vi "Check If Custom Device Enabled.vi"(8 "error in (no error)":errorcluster, 11 "Ballard ARINC 429 ref":T1 format="%.0x") -> (0 "error out":errorcluster, 2 "Is Custom Device Enabled?":bool, 3 "Ballard ARINC 429 ref":T1 format="%.0x")   [LabVIEW 2020, in "Ballard ARINC 429 Scripting.lvlib"]
doc: "Returns a boolean value that is <b>True</b> if the Ballard ARINC 429 custom device is <b>Enabled</b>, and <b>False</b> if it is <b>Disabled</b>."
uses:
  Ballard ARINC 429 Scripting.lvlib
  <vilib>/NI VeriStand/Custom Device API/Custom Device Item Ref.ctl
  Constants.vi
  <vilib>/NI VeriStand/Custom Device API/Custom Device API.lvlib
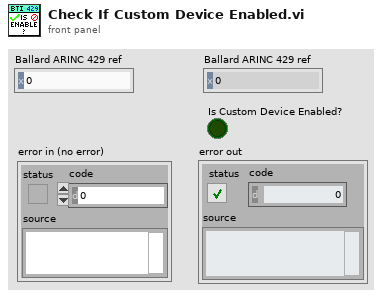
[diagram p1: front panel]
types:
  T1 = typedef "Custom Device API.lvlib/Custom Device Item Ref.ctl" = u64
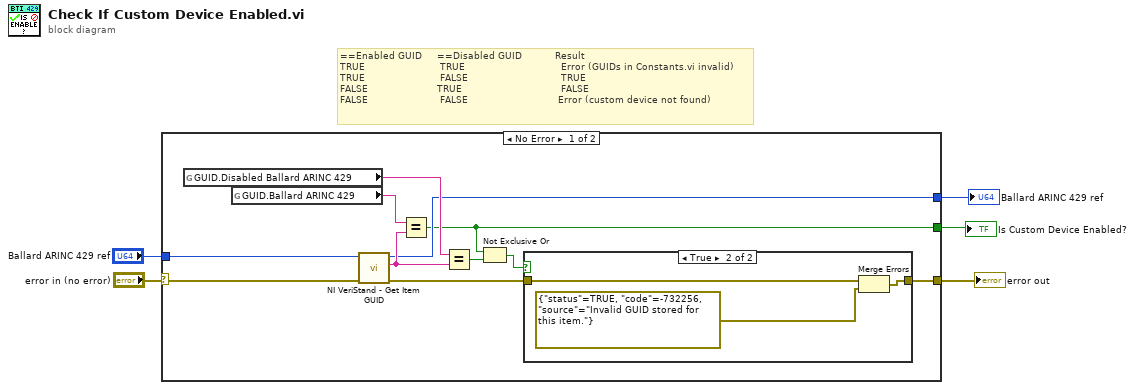
[diagram p0: block diagram]
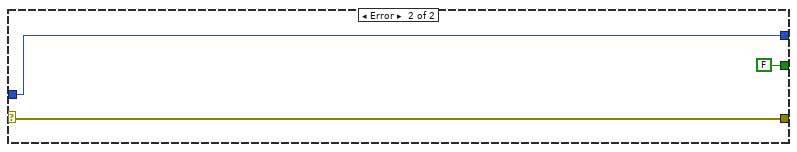
[diagram p3: hidden frame]
diagram:
  # "==Enabled GUID     ==Disabled GUID           Result\nTRUE                         TRUE                                Error (GUIDs in Constants.vi invalid)\nTRUE                         FALSE                               TRUE\nFALSE                       TRUE                                 FALSE\nFALSE                        FALSE                              Error (custom device not found)"
  n1 = case shown="No Error" "error in (no error)" {
    selector: "error in (no error)" -> [w12 w22]
    tunnel: "Ballard ARINC 429 ref" -> [w15 w21]
    tunnel: [w10 w22] -> w2
    tunnel: [w7 FALSE] -> w3
    tunnel: [w9 w21] -> w1
    frame No Error {
      n2 = global read "Constants.vi" "GUID.Disabled Ballard ARINC 429"() -> (w13:string)
      n3 = global read "Constants.vi" "GUID.Ballard ARINC 429"() -> (w16:string)
      n4 = call <vilib>:"NI VeriStand - Get Item GUID.vi"("error in (no error)"=w12, "Item Ref in"=w15) -> ("error out"=w11:errorcluster, "GUID"=w14:string, "Item Ref out"=w9:T1)  [unwired: 7 in]
      n5 = Equal?(x=w16, y=w14) -> (x = y?=w7:bool)
      n6 = Equal?(x=w13, y=w14) -> (x = y?=w8:bool)
      n7 = Not Exclusive Or(1:w8, 2:w7) -> (0:w6:bool)
      n8 = case shown="True" w6 {
        tunnel: [w17 w18] -> w10
        tunnel: w11 -> [w17 w20]
        frame False {
        }
        frame True {
          n9 = Merge Errors(w20, errorcluster {"status"=TRUE, "code"=-732256, "source"="Invalid GUID stored for this item."} ("New Error")) -> (w18:errorcluster)
        }
      }
    }
    frame Error {
    }
  }
  "Is Custom Device Enabled?" <- w3
  "error out" <- w2
  "Ballard ARINC 429 ref" <- w1
